vi "AttackHim.vi"(8 "error in (no error)":errorcluster, 9 "Cube":i32, 10 "Rival":refnum<class "Peasant.lvclass">, 11 "Peasant in":refnum<class "Peasant.lvclass">) -> (0 "error out":errorcluster, 1 "CurrentAttack":i32, 2 "Rival out":refnum<class "Peasant.lvclass">, 3 "Peasant out":refnum<class "Peasant.lvclass">)   [LabVIEW 2021, in "Peasant.lvclass"]
uses:
  Peasant.lvclass
  Peasant.lvclass/Peasant.ctl
  Read Peasant Attributes.vi
  Write Peasant Attributes.vi
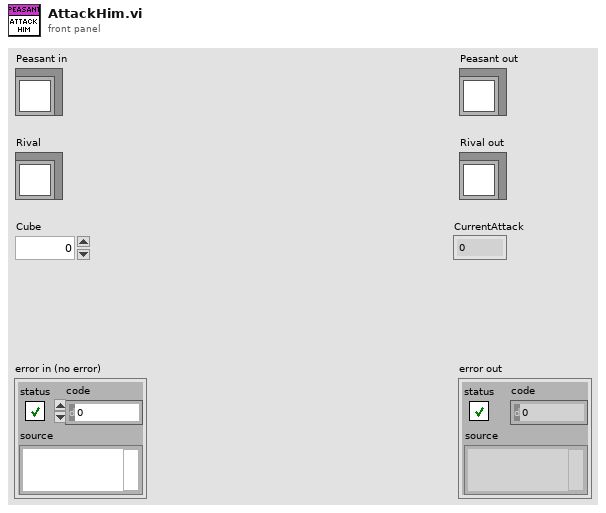
[diagram p1: front panel]
types:
  T1 = typedef "PeasantCluster.ctl" = cluster{"Health":i32, "Stamina":i32, "Attack":i32, "Defense":i32, "Sing":i32}
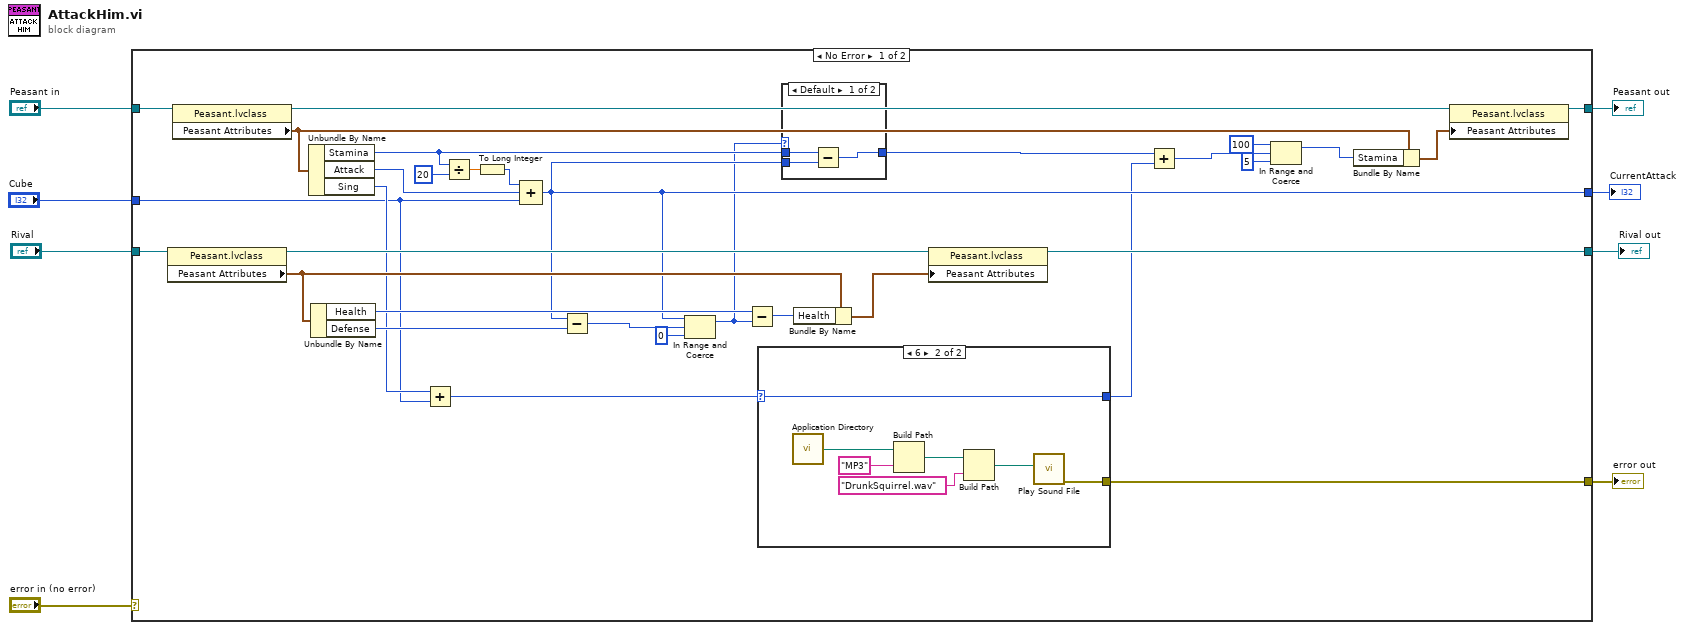
[diagram p0: block diagram]
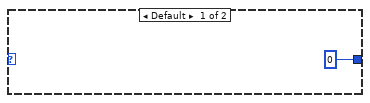
[diagram p3: hidden frame]
diagram:
  n1 = case shown="No Error" "error in (no error)" {
    selector: "error in (no error)" -> [_ w55]
    tunnel: [w25 w55] -> w7
    tunnel: [w26 w54] -> w5
    tunnel: "Peasant in" -> [w40 w54]
    tunnel: "Rival" -> [w39 w53]
    tunnel: "Cube" -> [w11 _]
    tunnel: [w33 w53] -> w2
    tunnel: [w15 _] -> w1
    frame No Error {
      n2 = property class="Peasant.lvclass"(reference=w39) -> (reference out=w35:refnum<class "Peasant.lvclass">, "Peasant Attributes"=w37:T1)  [unwired: 1 in, 1 out]
      n3 = property class="Peasant.lvclass"(reference=w40) -> (reference out=w29:refnum<class "Peasant.lvclass">, "Peasant Attributes"=w28:T1)  [unwired: 1 in, 1 out]
      n4 = Unbundle By Name(w28) -> ("Stamina"=w19:i32, "Attack"=w20:i32, "Sing"=w12:i32)
      n5 = Unbundle By Name(w37) -> ("Health"=w38:i32, "Defense"=w32:i32)
      n6 = Add(x=w12, y=w11) -> (x+y=w10:i32)
      n7 = Divide(x=w19, y=20) -> (x/y=w17:dbl)
      n8 = To Long Integer(number=w17) -> (32bit integer=w16:i32)
      n9 = Compound Arithmetic op=ADD(w16, w20, w11) -> (w15:i32)
      n10 = Subtract(x=w15, y=w32) -> (x-y=w30:i32)
      n11 = In Range and Coerce(upper limit=w15, x=w30, lower limit=0) -> (coerced(x)=w13:i32)  [unwired: 1 out]
      n12 = Subtract(x=w38, y=w13) -> (x-y=w36:i32)
      n13 = case shown="6" w10 {
        selector: w10 -> [_ w46]
        tunnel: [_ w47] -> w25
        tunnel: [0 w46] -> w9
        frame Default {
        }
        frame 6 {
          n14 = call <vilib>:"Application Directory.vi"() -> ("Application Directory"=w52:path)
          n15 = Build Path(base path=w52, name or relative path="MP3") -> (appended path=w50:path)
          n16 = Build Path(base path=w50, name or relative path="DrunkSquirrel.wav") -> (appended path=w48:path)
          n17 = call <vilib>:"Play Sound File.vi"("path"=w48) -> ("error out"=w47:errorcluster)  [unwired: 9 in, 1 out]
        }
      }
      n18 = case shown="Default" w13 {
        tunnel: [w43 w44] -> w24
        tunnel: w19 -> [w42 w44]
        tunnel: w15 -> [w41 _]
        frame Default {
          n19 = Subtract(x=w42, y=w41) -> (x-y=w43:i32)
        }
        frame 0 {
        }
      }
      n20 = Bundle By Name(cluster=w37, "Health"=w36) -> (w34:T1)
      n21 = property class="Peasant.lvclass"(reference=w35, "Peasant Attributes"=w34) -> (reference out=w33:refnum<class "Peasant.lvclass">)  [unwired: 1 in, 1 out]
      n22 = Add(x=w24, y=w9) -> (x+y=w23:i32)
      n23 = In Range and Coerce(upper limit=100, x=w23, lower limit=5) -> (coerced(x)=w21:i32)  [unwired: 1 out]
      n24 = Bundle By Name(cluster=w28, "Stamina"=w21) -> (w27:T1)
      n25 = property class="Peasant.lvclass"(reference=w29, "Peasant Attributes"=w27) -> (reference out=w26:refnum<class "Peasant.lvclass">)  [unwired: 1 in, 1 out]
    }
    frame Error {
    }
  }
  "error out" <- w7
  "Peasant out" <- w5
  "Rival out" <- w2
  "CurrentAttack" <- w1
